vi "总磷氨氮公式读取_N.vi"(8 "error in (no error)":errorcluster caption="错误输入（无错误）", 9 "量程":enum16{"低量程", "高量程"}(ring), 10 "测量模式":enum16{"水样测量", "空白核查", "跨度核查", "标样核查", "加标回收"}(ring), 11 "测量参数":enum16{"氨氮", "总磷"}(ring)) -> (0 "error out":errorcluster caption="错误输出", 3 "公式":cluster{"X^2":dbl, "X":dbl, "b":dbl})   [LabVIEW 2016]
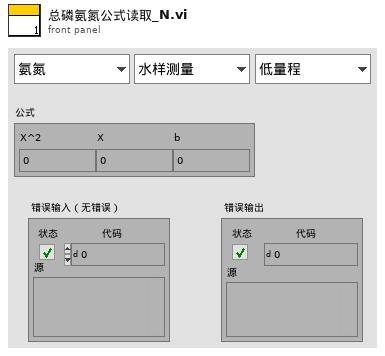
[diagram p1: front panel]
types:
  T1 = cluster{"FLOAT[0]":sgl, "FLOAT[1]":sgl, "FLOAT[2]":sgl}
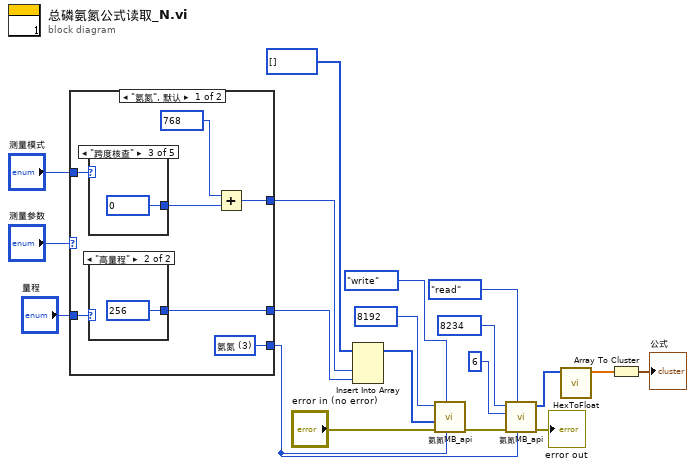
[diagram p0: block diagram]
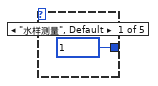
[diagram p2: hidden frame]
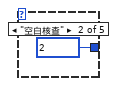
[diagram p3: hidden frame]
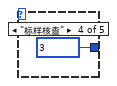
[diagram p4: hidden frame]
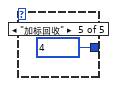
[diagram p5: hidden frame]
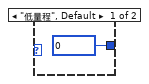
[diagram p6: hidden frame]
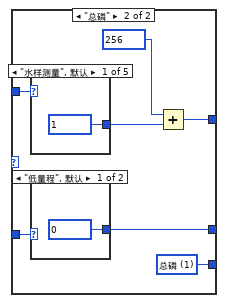
[diagram p7: hidden frame]
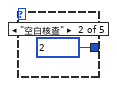
[diagram p8: hidden frame]
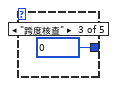
[diagram p9: hidden frame]
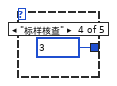
[diagram p10: hidden frame]
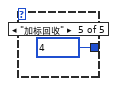
[diagram p11: hidden frame]
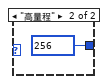
[diagram p12: hidden frame]
diagram:
  n1 = case shown="\"氨氮\", 默认" "测量参数" {
    tunnel: "测量模式" -> [w24 w38]
    tunnel: "量程" -> [w25 w39]
    tunnel: [w26 w40] -> w5
    tunnel: [w20 w34] -> w9
    tunnel: [w23 w37] -> w8
    frame "氨氮", Default {
      w26 = u16 3 items=["总磷"=1, "氨氮"=3] ("站号")
      n2 = case shown="\"跨度核查\"" w24 {
        tunnel: [u16 1 ("starting address") u16 2 ("starting address") u16 0 ("starting address") u16 3 ("starting address") u16 4 ("starting address")] -> w22
        frame "水样测量", Default {
        }
        frame "空白核查" {
        }
        frame "跨度核查" {
        }
        frame "标样核查" {
        }
        frame "加标回收" {
        }
      }
      n3 = case shown="\"高量程\"" w25 {
        tunnel: [u16 0 ("starting address") u16 256 ("starting address")] -> w23
        frame "低量程", Default {
        }
        frame "高量程" {
        }
      }
      n4 = Add(x=u16 768 ("starting address"), y=w22) -> (x+y=w20:u16)
    }
    frame "总磷" {
      w40 = u16 1 items=["总磷"=1, "氨氮"=3] ("站号")
      n5 = case shown="\"水样测量\", 默认" w38 {
        tunnel: [u16 1 ("starting address") u16 2 ("starting address") u16 0 ("starting address") u16 3 ("starting address") u16 4 ("starting address")] -> w36
        frame "水样测量", Default {
        }
        frame "空白核查" {
        }
        frame "跨度核查" {
        }
        frame "标样核查" {
        }
        frame "加标回收" {
        }
      }
      n6 = case shown="\"低量程\", 默认" w39 {
        tunnel: [u16 0 ("starting address") u16 256 ("starting address")] -> w37
        frame "低量程", Default {
        }
        frame "高量程" {
        }
      }
      n7 = Add(x=u16 256 ("starting address"), y=w36) -> (x+y=w34:u16)
    }
  }
  n8 = Insert Into Array(array=u16[] [] ("数组"), new element #1=w9, new element #2=w8) -> (w1:u16[])  [unwired: 1 in]
  n9 = call "氨氮MB_api.vi"("Slave ID"=w5, "STEP"=enum16{"open", "read", "write", "close"}."write", "Error in"="error in (no error)", "values"=w1, "starting address"=u16 8192) -> ("error out"=w4:errorcluster)  [unwired: 3 in, 3 out]
  n10 = call "氨氮MB_api.vi"("Slave ID"=w5, "STEP"=enum16{"open", "read", "write", "close"}."read", "Error in"=w4, "quantity"=u16 6, "starting address"=u16 8234) -> ("error out"=→"error out":errorcluster, "Registers"=w15:u16[])  [unwired: 3 in, 2 out]
  n11 = call "HexToFloat.vi"("数组"=w15) -> ("FLOAT"=w14:sgl[])  [unwired: 10 in]
  n12 = Array To Cluster(array=w14) -> (cluster=→"公式":T1)
